vi "WPI_CameraSend Images To PC Loop.vi"(10 "BackCameraDevRef":T1, 11 "FrontCameraDevRef":T1) -> ()   [LabVIEW 2018]
uses:
  <vilib>/Rock Robotics/WPI/Camera/WPI_CameraDevRef.ctl
  <vilib>/Rock Robotics/SystemInterfaces/NetworkCommunication/NetComm_UsageReport_ResourceType.ctl
  Framework/Robot Global Data.vi
panel:
  in  "error in (no error)":errorcluster
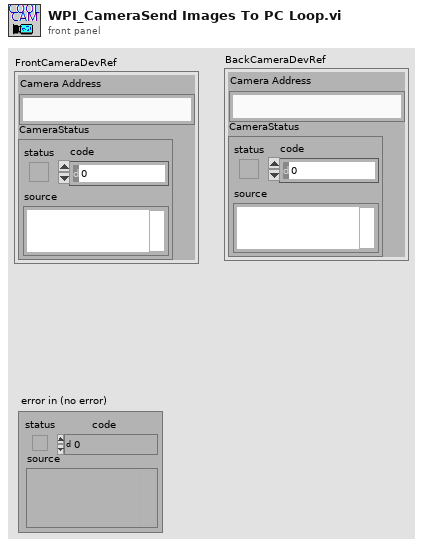
[diagram p1: front panel]
types:
  T1 = typedef "WPI_CameraDevRef.ctl" = cluster{"Camera Address":string, "CameraStatus":errorcluster}
  T2 = cluster{"fps":i32, "compression":i32, "compression 2":i32}
  T3 = typedef "NetComm_UsageReport_ResourceType.ctl" = enum8{"Controller", "Module", "Language", "CANPlugin", "Accelerometer", "ADXL345", "AnalogChannel", "AnalogTrigger", "AnalogTriggerOutput", "CANJaguar", "Compressor", "Counter", "Dashboard", "DigitalInput", "DigitalOutput", "DriverStationCIO", "DriverStationEIO", "DriverStationLCD", "Encoder", "GearTooth", "Gyro", "I2C", "Framework", "Jaguar", "Joystick", "Kinect", "KinectStick", "PIDController", "Preferences", "PWM", "Relay", "RobotDrive", "SerialPort", "Servo", "Solenoid", "SPI", "Task", "Ultrasonic", "Victor", "Button", "Command", "AxisCamera", "PCVideoServer", "SmartDashboard", "Talon", "HiTechnicColorSensor", "HiTechnicAccel", "HiTechnicCompass", "SRF08", "AnalogOutput", "Victor SP", "Talon SRX", "CAN Talon SRX", "ADXL362 Accel", "ADXRS450 Gyro", "Rev SPARK", "Mindsensors SD540", "Digital Filter", "ADIS16448", "PDP", "PCM", "PigeonIMU", "Nidec Brushless", "CTRE CANifier", "CTRE Future 0", "CTRE Future 1", "CTRE Future 2", "CTRE Future 3", "CTRE Future 4", "CTRE Future 5", "CTRE Future 6", "Linear Filter", "Xbox Controller", "USB Camera", "NavX", "Pixy", "Pixy2", "ScanseSweep", "Shuffleboard", "CAN", "Digilent DMC60", "PWM Victor SPX", "Rev SPARK MAX PWM", "Rev SPARK MAX CAN", "ADIS16470"}
  T4 = enum16{"Update Mode", "Get Image", "Get Image Data"}
  T5 = typedef "Image Type" = u32
  T6 = typedef "IMAQ Image.ctl" = refnum<image>
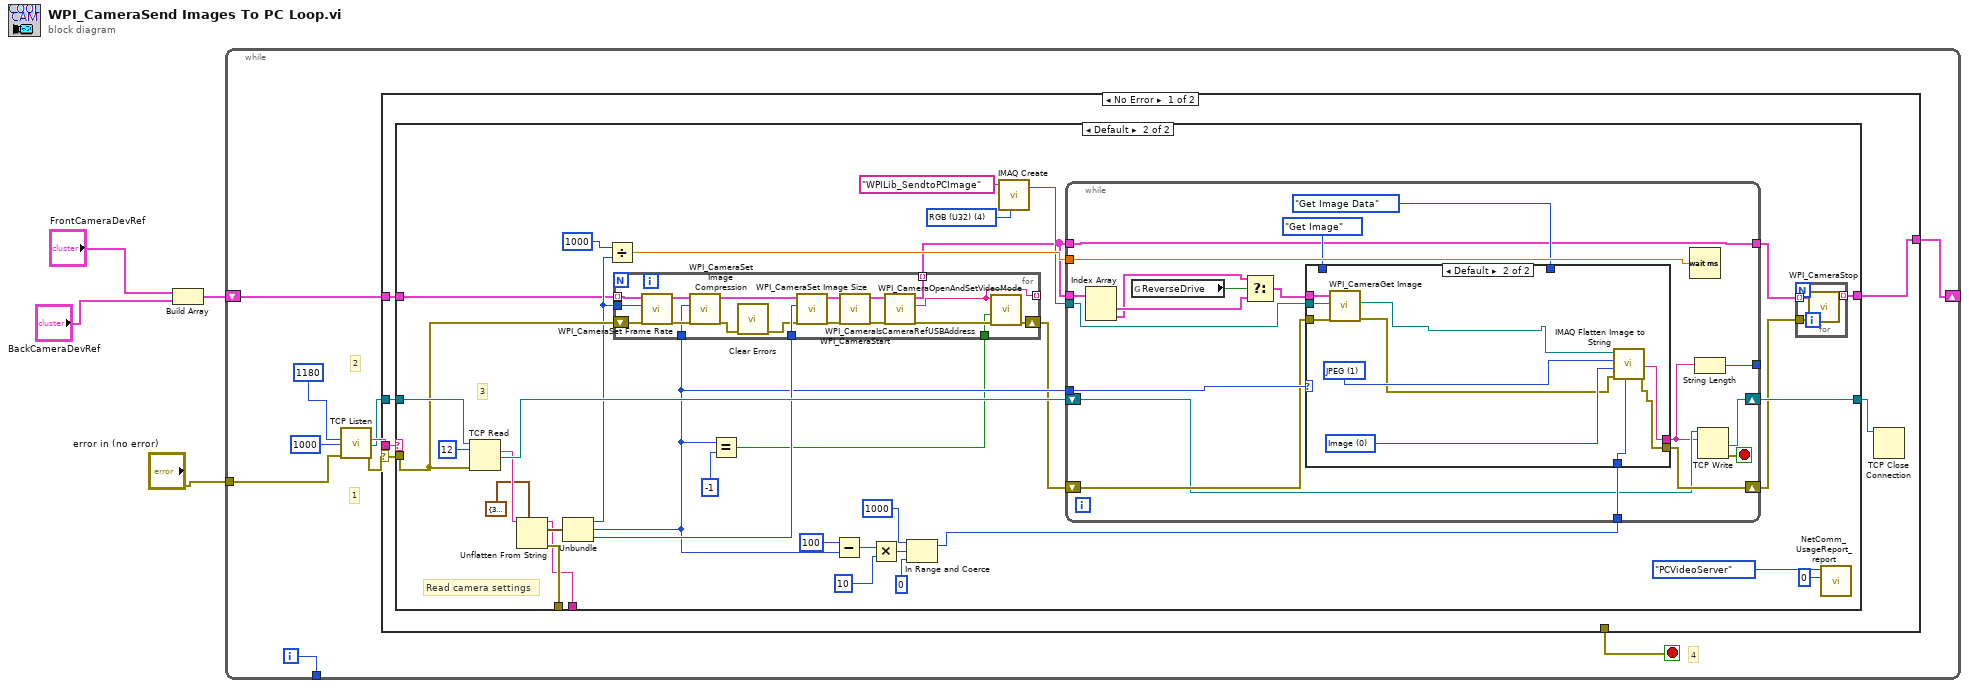
[diagram p0: block diagram]
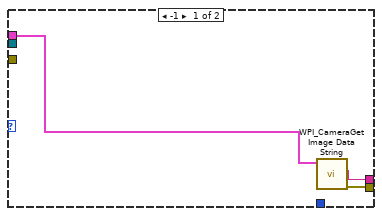
[diagram p3: hidden frame]
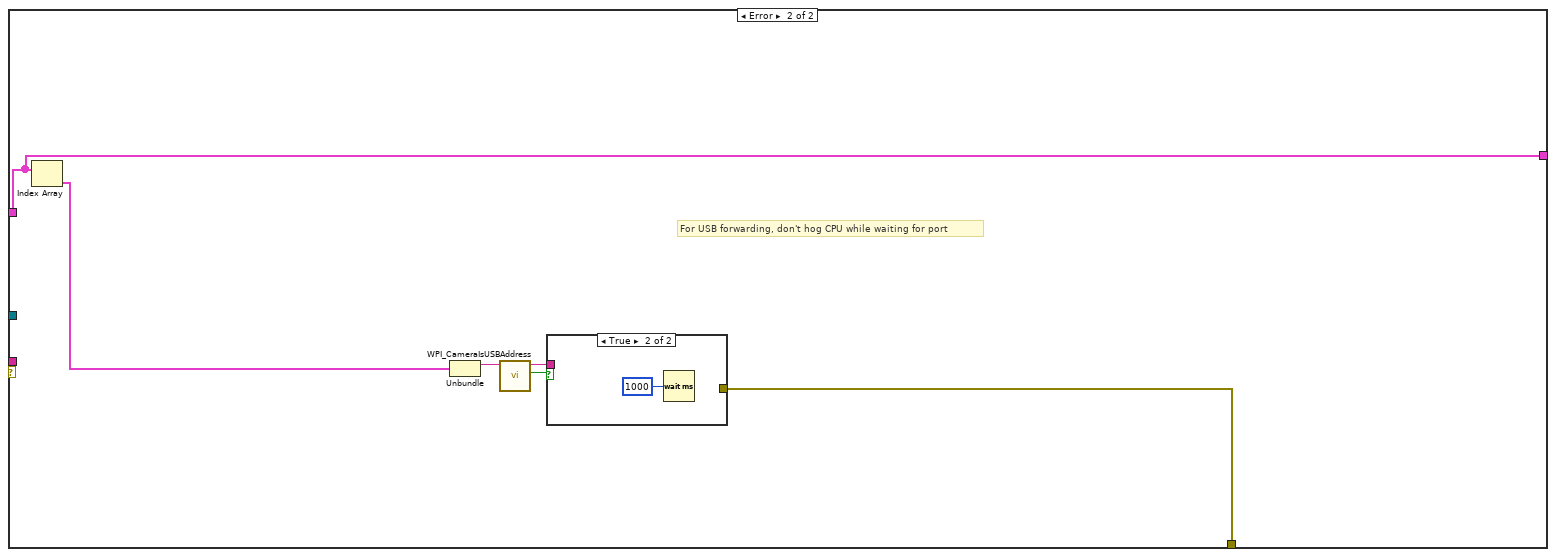
[diagram p4: hidden frame]
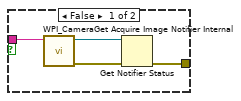
[diagram p5: hidden frame]
diagram:
  n1 = Build Array("FrontCameraDevRef", "BackCameraDevRef") -> (w1:T1[])
  n2 = while {
    tunnel: "error in (no error)" -> [w13]
    tunnel: [w7] -> _
    shift-right: [w5] -> _
    shift-left: w1 -> [w6]
    i -> [w7]
    stop <- w11 stop-if-true
    # "4"
    # "1"
    # "2"
    n3 = call <vilib>:"TCP Listen.vi"("error in (no error)"=w13, "timeout ms (wait forever: -1)"=u16 1000 ("port"), "port"=u16 1180) -> ("error out"=w9:errorcluster, "remote address"=w14:string, "connection ID"=w12:refnum<k5>)  [unwired: 1 in, 5 out]
    n4 = case shown="No Error" w9 {
      selector: w9 -> [w17 _]
      tunnel: w14 -> [w20 _]
      tunnel: w12 -> [w19 _]
      tunnel: [_ w117] -> w11
      tunnel: w6 -> [w16 w112]
      tunnel: [w15 w112] -> w5
      frame No Error {
        n5 = case shown="Default" w20 {
          tunnel: w17 -> [_ w47]
          tunnel: w19 -> [w22 w51]
          tunnel: [w22 w57] -> w18
          tunnel: [_ w30] -> _
          tunnel: [_ w29] -> _
          tunnel: w16 -> [w21 w26]
          tunnel: [w21 w24] -> w15
          frame "localhost" {
          }
          frame Default {
            w52 = T5 4 items=["Grayscale (U8)", "Grayscale (I16)", "Grayscale (SGL)", "Complex (CSG)", "RGB (U32)", "HSL (U32)", "RGB (U64)", "Grayscale (U16)"] ("Image Type")
            # "Read camera settings"
            # "3"
            n6 = TCP Read(connection ID=w51, bytes to read=12, error in (no error)=w47) -> (connection ID out=w50:refnum<k5>, data out=w48:string)  [unwired: 2 in, 1 out]
            n7 = Unflatten From String(type=T2 {"fps"=30, "compression"=32, "compression 2"=32} ("Camera Settings"), binary string=w48) -> (rest of the binary string=w29:string, value=w46:T2, error out=w30:errorcluster)  [unwired: 3 in]
            n8 = Unbundle(w46) -> ("fps"=w43:i32, "compression"=w32:i32, "compression 2"=w45:i32)
            n9 = Divide(x=u16 1000 ("port"), y=w43) -> (x/y=w42:dbl)
            n10 = Equal?(x=w32, y=-1) -> (x = y?=w31:bool)
            n11 = for {
              tunnel: [w79] -> _ mode=indexing
              tunnel: [w75] -> w23 mode=indexing
              tunnel: w45 -> [w68]
              tunnel: w43 -> [w67]
              tunnel: w32 -> [w66]
              tunnel: w31 -> [w65]
              shift-right: [w62] -> w27
              shift-left: w47 -> [w71]
              tunnel: w26 -> [w61] mode=indexing
              n12 = call <vilib>:"WPI_CameraSet Frame Rate.vi"("error in (no error)"=w71, "Frame Rate (fps)"=w67, "CameraDevRef"=w61) -> ("error out"=w70:errorcluster, "CameraDevRef Out"=w74:T1)  [unwired: 7 in]
              n13 = call <vilib>:"WPI_CameraSet Image Compression.vi"("error in (no error)"=w70, "Compression"=w66, "CameraDevRef"=w74) -> ("error out"=w64:errorcluster, "CameraDevRef Out"=w73:T1)  [unwired: 7 in]
              n14 = call <vilib>:"Clear Errors.vi"("error in (no error)"=w64) -> ("error out"=w63:errorcluster)  [unwired: 5 in, 1 out]
              n15 = call <vilib>:"WPI_CameraSet Image Size.vi"("error in (no error)"=w63, "Image Size"=w68, "CameraDevRef"=w73) -> ("error out"=w69:errorcluster, "CameraDevRef Out"=w72:T1)  [unwired: 7 in]
              n16 = call <vilib>:"WPI_CameraStart.vi"("error in (no error)"=w69, "CameraDevRef"=w72) -> ("error out"=w78:errorcluster, "CameraDevRef"=w76:T1)  [unwired: 8 out]
              n17 = call <vilib>:"WPI_CameraIsCameraRefUSBAddress.vi"("error in (no error)"=w78, "CameraDevRef"=w76) -> ("error out"=w77:errorcluster, "Camera Address Out"=w79:string, "CameraDevRef out"=w75:T1)  [unwired: 6 in, 1 out]
              n18 = call <vilib>:"WPI_CameraOpenAndSetVideoMode.vi"("error in (no error)"=w77, "USB JPEG"=w65, "Camera Address"=w79) -> ("error out"=w62:errorcluster)  [unwired: 8 in]
            }
            n19 = Subtract(x=100, y=w32) -> (x-y=w37:i32)
            n20 = Multiply(x=w37, y=10) -> (x*y=w39:i32)
            n21 = In Range and Coerce(upper limit=1000, x=w39, lower limit=0) -> (coerced(x)=w35:i32)  [unwired: 1 out]
            n22 = call "IMAQ Create"("Image Name"="WPILib_SendtoPCImage", "Image Type"=w52) -> ("New Image"=w28:T6)  [unwired: 3 in, 1 out]
            n23 = while {
              tunnel: w23 -> [w91]
              shift-right: [w81] -> w57
              shift-left: w50 -> [w84]
              tunnel: w28 -> [w98]
              tunnel: [w85] -> w56
              tunnel: w23 -> [w85]
              tunnel: w35 -> [w97]
              tunnel: w42 -> [w96]
              tunnel: [w95] -> _
              tunnel: w32 -> [w94]
              shift-right: [w86] -> w25
              shift-left: w27 -> [w87]
              stop <- w82 stop-if-true
              n24 = Index Array(array=w91) -> (element #1=w90:T1, element #2=w89:T1)  [unwired: 2 in]
              n25 = global read "Robot Global Data.vi" "ReverseDrive"() -> (w80:bool)
              n26 = Select(t=w89, s=w80, f=w90) -> (s? t:f=w88:T1)
              n27 = case shown="Default" w94 {
                tunnel: [w100 w111] -> w83
                tunnel: w88 -> [w101 w106]
                tunnel: w98 -> [_ w105]
                tunnel: w97 -> [_ w108]
                tunnel: [w99 w107] -> w86
                tunnel: T4."Get Image Data" ("Operation") -> [_ _]
                tunnel: T4."Get Image" ("Operation") -> [_ _]
                tunnel: w87 -> [_ w104]
                frame -1 {
                  n28 = call <vilib>:"WPI_CameraGet Image Data String.vi"("CameraDevRef"=w101) -> ("error out"=w99:errorcluster, "Image Data String"=w100:string)  [unwired: 8 in, 1 out]
                }
                frame Default {
                  w109 = 0 items=["Image", "Image and Vision Info", "Reference to Image"] ("Type of Flatten (Image and Vision Info)")
                  w110 = 1 items=["None", "JPEG", "PACKED BINARY"] ("Compression (None)")
                  n29 = call <vilib>:"WPI_CameraGet Image.vi"("error in (no error)"=w104, "Image"=w105, "CameraDevRef"=w106) -> ("error out"=w103:errorcluster, "Image Out"=w102:T6)  [unwired: 6 in, 1 out]
                  n30 = call "IMAQ Flatten Image to String"("Quality (750)"=w108, "error in (no error)"=w103, "Type of Flatten (Image and Vision Info)"=w109, "Compression (None)"=w110, "Image"=w102) -> ("error out"=w107:errorcluster, "Data String"=w111:string)  [unwired: 5 in]
                }
              }
              n31 = Wait (ms)(milliseconds to wait=w96) -> ()  [unwired: 1 out]
              n32 = String Length(string=w83) -> (length=w95:i32)
              n33 = TCP Write(connection ID=w84, data in=w83) -> (connection ID out=w81:refnum<k5>, error out=w82:errorcluster)  [unwired: 2 in, 1 out]
            }
            n34 = for {
              tunnel: w56 -> [w60] mode=indexing
              tunnel: w25 -> [w59]
              tunnel: [w58] -> w24 mode=indexing
              n35 = call <vilib>:"WPI_CameraStop.vi"("error in (no error)"=w59, "CameraDevRef"=w60) -> ("CameraDevRef"=w58:T1)  [unwired: 9 out]
            }
            n36 = call <vilib>:"NetComm_UsageReport_report.vi"("Instance Number"=u8 0, "Resource Type"=NetComm_UsageReport_ResourceType."PCVideoServer") -> ()  [unwired: 10 in]
          }
        }
        n37 = TCP Close Connection(connection ID=w18) -> ()  [unwired: 1 in, 3 out]
      }
      frame Error {
        # "For USB forwarding, don't hog CPU while waiting for port"
        n38 = Index Array(array=w112) -> (element=w114:T1)  [unwired: 1 in]
        n39 = Unbundle(w114) -> ("Camera Address"=w113:string)  [unwired: 1 out]
        n40 = call <vilib>:"WPI_CameraIsUSBAddress.vi"("Camera Address In"=w113) -> ("USB?"=w115:bool, "Camera Address Out"=w116:string)  [unwired: 8 in, 1 out]
        n41 = case shown="True" w115 {
          tunnel: [w121 _] -> w117
          tunnel: w116 -> [w118 _]
          frame False {
            n42 = call <vilib>:"WPI_CameraGet Acquire Image Notifier Internal.vi"("Camera Address"=w118) -> ("error out"=w119:errorcluster, "Acquire Image Notifier"=w120:refnum<notifier>)  [unwired: 1 in, 8 out]
            n43 = Get Notifier Status(notifier=w120, error in (no error)=w119) -> (error out=w121:errorcluster)  [unwired: 4 out]
          }
          frame True {
            n44 = Wait (ms)(milliseconds to wait=u32 1000) -> ()  [unwired: 1 out]
          }
        }
      }
    }
  }
